vi "About control creator.vi"   [LabVIEW 2013]
uses:
  Dialog/MessageBox/pictures/pictures.ctl
  Dialog/MessageBox/MessageBox.lvclass
types:
  T1 = typedef "pictures.ctl" = enum16{"Alarm", "Download", "Edition", "Encrypted", "Error", "Hardware Information", "Important", "Memory", "Network", "Package", "Password", "Readme", "Search", "System", "USB", "User", "Wireless", "www"}
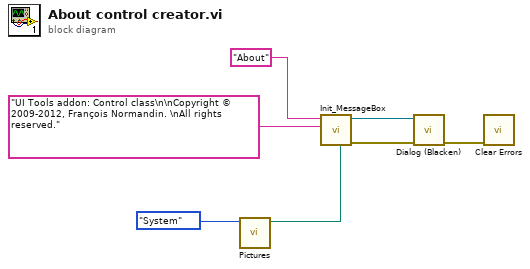
[diagram p0: block diagram]
diagram:
  n1 = call "Pictures.vi"("Pictures"=pictures."System") -> ("Path"=w6:path)  [unwired: 10 out]
  n2 = call "Init_MessageBox.vi"("Image path"=w6, "Message"="UI Tools addon: Control class\n\nCopyright © 2009-2012, François Normandin. \nAll rights reserved." ("MsgBox Title"), "MsgBox Title"="About") -> ("error out"=w2:errorcluster, "MessageBox out"=w3:refnum<class "MessageBox.lvclass">)  [unwired: 4 in, 3 out]
  n3 = call-dynamic "Dialog (Blacken).vi"("error in (no error)"=w2, "Dialog in"=w3) -> ("error out"=w1:errorcluster)  [unwired: 1 in, 8 out]
  n4 = call <vilib>:"Clear Errors.vi"("error in (no error)"=w1) -> ()  [unwired: 7 out]
